vi "publishLFOA.vi"(8 "error in (no error)":errorcluster, 9 "Byte_Size":i32, 10 "Path":string, 11 "ElectrometerController in":refnum<class "ElectrometerController.lvclass">) -> (0 "error out":errorcluster, 3 "ElectrometerController out":refnum<class "ElectrometerController.lvclass">)   [LabVIEW 2016, in "ElectrometerController.lvclass"]
uses:
  ElectrometerController.lvclass
  ts_sallv_calibrationelectrometer/DataTypes/logevent_LargeFileObjectAvailable.ctl
  ElectrometerController.lvclass/ElectrometerController.ctl
  ts_electrometeruserevents/PubSubDataEvent/PubSubDataEvent.lvclass/PubSubDataEvent.ctl
  ts_sallv_calibrationelectrometer/SALLV_calibrationElectrometer.lvlib
  ts_electrometeruserevents/PubSubDataEvent/PubSubDataEvent.lvclass
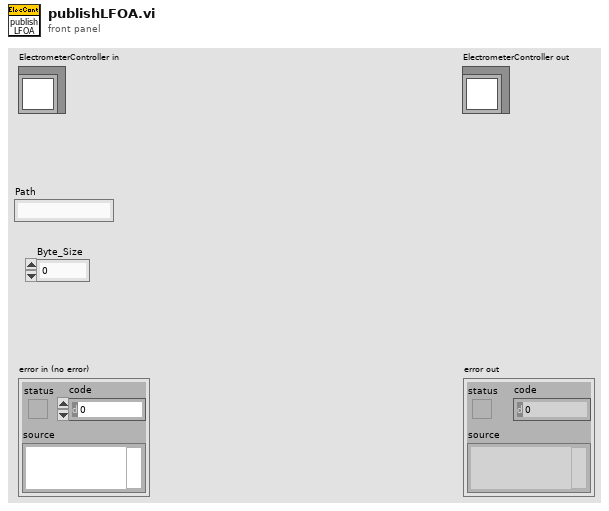
[diagram p1: front panel]
types:
  T1 = typedef "SALLV_calibrationElectrometer.lvlib/logevent_LargeFileObjectAvailable.ctl" = cluster{"URL":string, "Generator":string, "Version":sgl, "Checksum":string, "Mime_Type":string, "Byte_Size":i32, "ID":string, "priority":i32}
  T2 = typedef "ElectrometerTypedefs.lvlib/PubDataEvents.ctl" = cluster{"DetailedState":refnum<user-event>, "ErrorCode":refnum<user-event>, "Heartbeat":refnum<user-event>, "LoopTime_ms":refnum<user-event>, "LoopTimeOutOfRange":refnum<user-event>, "RejectedCommand":refnum<user-event>, "SummaryState":refnum<user-event>, "Timestamp":refnum<user-event>, "AppliedSettingsMatchStart":refnum<user-event>, "InternalState":refnum<user-event>, "MeasureRange":refnum<user-event>, "DigitalFilterChange":refnum<user-event>, "IntensityReq":refnum<user-event>, "MeasureType":refnum<user-event>, "Intensity":refnum<user-event>, "IntegrationTime":refnum<user-event>, "SettingsAppliedSerialConfiguration":refnum<user-event>, "SettingsAppliedReadingSettings":refnum<user-event>, "SettingVersions":refnum<user-event>, "LargeFileObjectAvailable":refnum<user-event>}
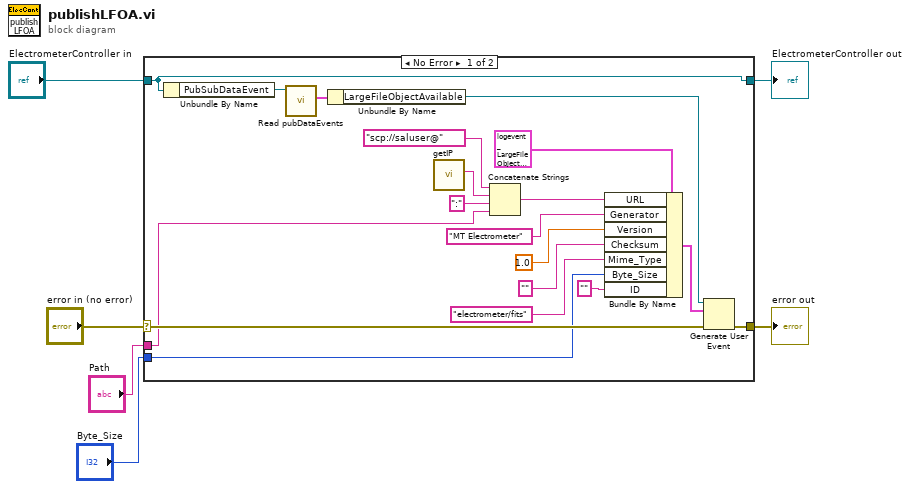
[diagram p0: block diagram]
diagram:
  n1 = case shown="No Error" "error in (no error)" {
    selector: "error in (no error)" -> [w24 w27]
    tunnel: [w23 w27] -> w5
    tunnel: [w25 w26] -> w3
    tunnel: "ElectrometerController in" -> [w25 w26]
    tunnel: "Path" -> [w20 _]
    tunnel: "Byte_Size" -> [w13 _]
    frame No Error {
      n2 = Unbundle By Name(w25) -> ("PubSubDataEvent"=w9:refnum<class "PubSubDataEvent.lvclass">)
      n3 = call "Read pubDataEvents.vi"("PubSubDataEvent in"=w9) -> ("pubDataEvents"=w8:T2)  [unwired: 9 in, 1 out]
      n4 = Unbundle By Name(w8) -> ("LargeFileObjectAvailable"=w7:refnum<user-event>)
      n5 = call "getIP.vi"() -> ("name"=w10:string)  [unwired: 9 in, 2 out]
      n6 = Concatenate Strings("scp://saluser@" ("string"), w10, ":" ("string"), w20) -> (w19:string)
      n7 = Bundle By Name(cluster=T1 {"URL"="", "Generator"="                                ", "Version"=0.0, "Checksum"="                                ", "Mime_Type"="                                ", "Byte_Size"=0, "ID"="                                ", "priority"=0} ("event data"), "URL"=w19, "Generator"="MT Electrometer", "Version"=sgl 1.0, "Checksum"="", "Mime_Type"="electrometer/fits" ("Mime"), "Byte_Size"=w13, "ID"="") -> (w21:T1)
      n8 = Generate User Event(user event=w7, event data cluster=w21, error in=w24) -> (error out=w23:errorcluster)  [unwired: 1 in, 1 out]
    }
    frame Error {
    }
  }
  "error out" <- w5
  "ElectrometerController out" <- w3
